vi "gwyscan refine path edges.vi"(0 "xypos":dbl[](array[numeric]), 1 "xypos_prev":dbl[](array[numeric]), 2 "zdata_prev":dbl[](array[numeric]), 3 "n_prev":i32, 4 "channel_prev":i32, 5 "threshold":dbl, 6 "xstep":dbl, 7 "error in (no error)":errorcluster, 8 "ystep":dbl, 9 "xreal":dbl, 10 "yreal":dbl, 11 "xoffset":dbl, 12 "yoffset":dbl) -> (20 "xypos OUT":dbl[](array[numeric]), 21 "xypos_prev OUT":dbl[](array[numeric]), 22 "zdata_prev OUT":dbl[](array[numeric]), 23 "function return":i32, 27 "error out":errorcluster)   [LabVIEW 2016, in "libgwyscan.lvlib"]
doc: "GWYSCANDLL_API int gwyscan_refine_path_edges(double* xypos, \n const double* xypos_prev, \n const double* zdata_prev, \n int n_prev, \n int channel_prev, \n double threshold, \n double xstep, \n double ystep, \n double xreal, \n double yreal, \n double xoffset, \n double yoffset);"
uses:
  libgwyscan.lvlib
  libgwyscan.dll
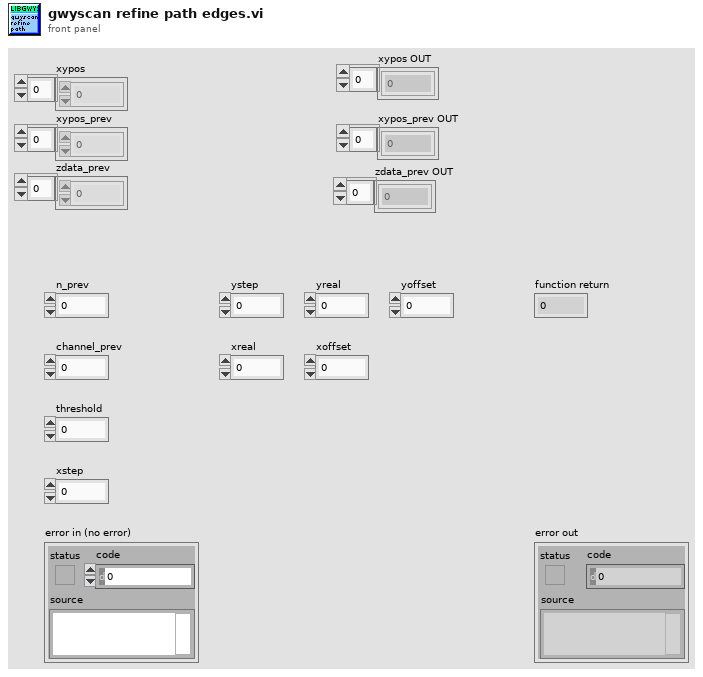
[diagram p1: front panel]
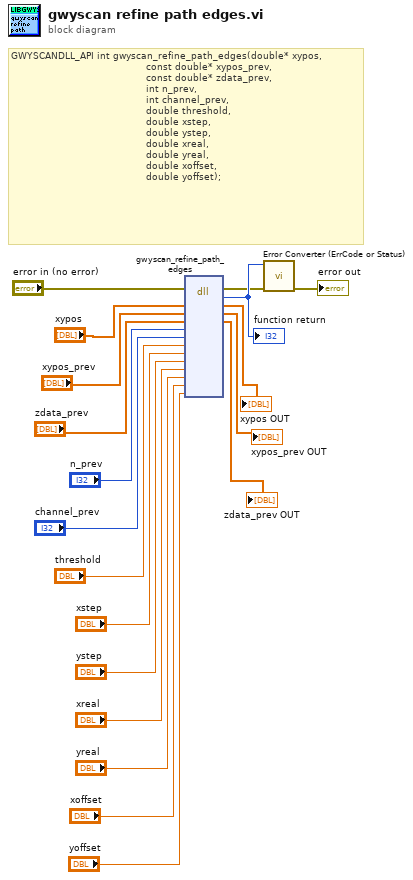
[diagram p0: block diagram]
diagram:
  # "GWYSCANDLL_API int gwyscan_refine_path_edges(double* xypos, \n                                             const double* xypos_prev, \n                                             const double* zdata_prev, \n                                             int n_prev, \n                                             int channel_prev, \n                                             double threshold, \n                                             double xstep, \n                                             double ystep, \n                                             double xreal, \n                                             double yreal, \n                                             double xoffset, \n                                             double yoffset);"
  n1 = dll-call lib="PTH2’abs CUsersCharlÃ¨ne BrillardDesktoplbni-lbniAFMController-BetaVersionv2.0.16-20190611 libgwyscan-1.2-labview2015-win32libgwyscan.dll" fn="gwyscan_refine_path_edges"(error in="error in (no error)", "xypos"="xypos", "xypos_prev"="xypos_prev", "zdata_prev"="zdata_prev", "n_prev"="n_prev", "channel_prev"="channel_prev", "threshold"="threshold", "xstep"="xstep", "ystep"="ystep", "xreal"="xreal", "yreal"="yreal", "xoffset"="xoffset", "yoffset"="yoffset") -> (error out=w5:errorcluster, "return type"=w19:i32, "xypos"=→"xypos OUT":dbl[], "xypos_prev"=→"xypos_prev OUT":dbl[], "zdata_prev"=→"zdata_prev OUT":dbl[])  [unwired: 11 in, 1 out]
  "function return" <- w19
  n2 = call "Error Converter (ErrCode or Status).vi"("error in (no error)"=w5, "error code"=w19) -> ("error out"=→"error out":errorcluster)  [unwired: 9 in]
